vi "Calculate Dynamic VariablesA.vi"(7 "Frequencies":dbl[](array[numeric]), 8 "Hours Under Test":dbl[](array[numeric]), 9 "Nom Freq":string) -> (0 "Agerate1Y":dbl, 1 "Agerate30D":dbl, 2 "C":dbl, 3 "B":dbl, 4 "RMS":dbl, 5 "A":dbl)   [LabVIEW 2024]
panel:
  out "Base ppm":dbl
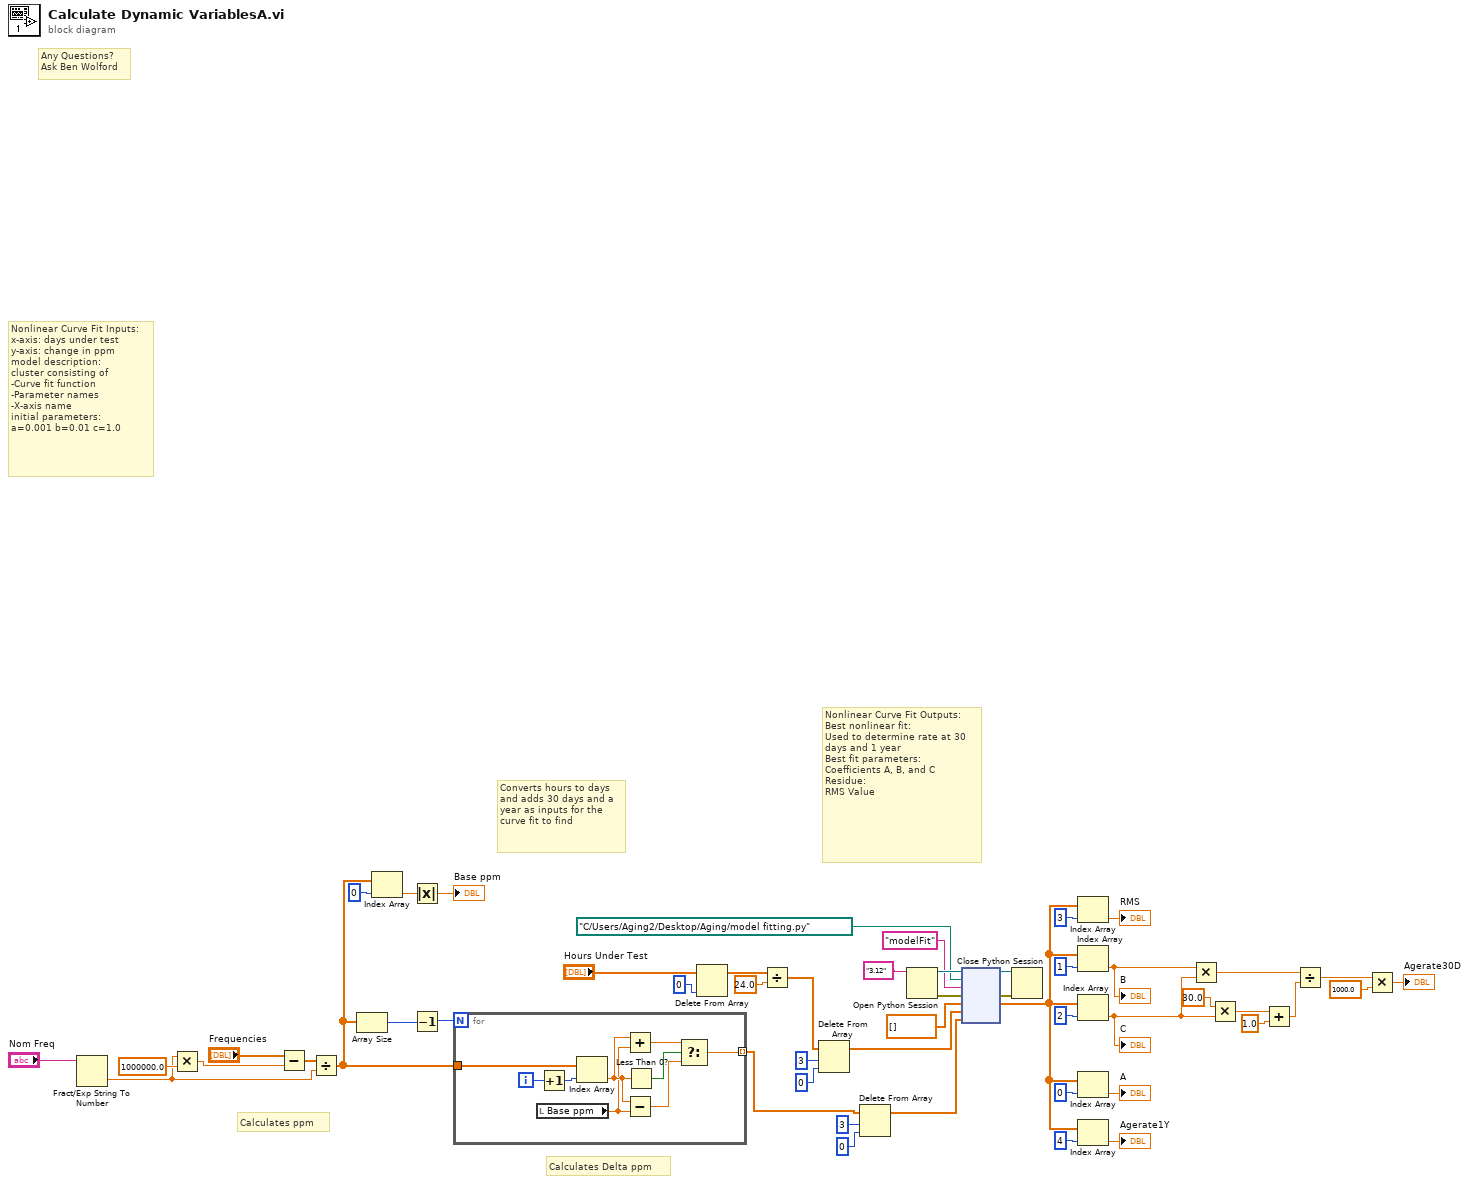
[diagram p0: block diagram]
diagram:
  # "Any Questions?\nAsk Ben Wolford"
  # "Calculates Delta ppm"
  # "Converts hours to days and adds 30 days and a year as inputs for the curve fit to find"
  # "Calculates ppm"
  # "Nonlinear Curve Fit Outputs:\nBest nonlinear fit:\nUsed to determine rate at 30 days and 1 year\nBest fit parameters:\nCoefficients A, B, and C\nResidue:\nRMS Value"
  # "Nonlinear Curve Fit Inputs:\nx-axis: days under test\ny-axis: change in ppm \nmodel description:\ncluster consisting of\n-Curve fit function\n-Parameter names\n-X-axis name\ninitial parameters:\na=0.001 b=0.01 c=1.0"
  n1 = Fract/Exp String To Number(string="Nom Freq") -> (number=w47:dbl)  [unwired: 3 in, 1 out]
  n2 = Multiply(x=w47, y=1000000.0) -> (x*y=w38:dbl)
  n3 = Subtract(x="Frequencies", y=w38) -> (x-y=w48:dbl[])
  n4 = Divide(x=w48, y=w47) -> (x/y=w43:dbl[])
  n5 = Array Size(array=w43) -> (size(s)=w45:i32)
  n6 = Index Array(array=w43, index=0) -> (element=w37:dbl)
  n7 = Absolute Value(x=w37) -> (abs(x)=→"Base ppm":dbl)
  n8 = Decrement(x=w45) -> (x-1=w44:i32)
  n9 = for {
    N: w44 -> [_]
    tunnel: w43 -> [w58]
    tunnel: [w55] -> w6 mode=indexing
    i -> [w59]
    n10 = local read "Base ppm"() -> (w53:dbl)
    n11 = Increment(x=w59) -> (x+1=w60:i32)
    n12 = Index Array(array=w58, index=w60) -> (element=w54:dbl)
    n13 = Add(x=w54, y=w53) -> (x+y=w52:dbl)
    n14 = Subtract(x=w54, y=w53) -> (x-y=w56:dbl)
    n15 = Less Than 0?(x=w54) -> (x < 0?=w57:bool)
    n16 = Select(t=w52, s=w57, f=w56) -> (s? t:f=w55:dbl)
  }
  n17 = Delete From Array(array="Hours Under Test", index=0) -> (array with subset deleted=w40:dbl[])  [unwired: 1 in, 1 out]
  n18 = Divide(x=w40, y=24.0) -> (x/y=w2:dbl[])
  n19 = Delete From Array(array=w2, length=3, index=0) -> (array with subset deleted=w1:dbl[])  [unwired: 1 out]
  n20 = Delete From Array(array=w6, length=3, index=0) -> (array with subset deleted=w5:dbl[])  [unwired: 1 out]
  n21 = Open Python Session(python version="3.12" ("Python version")) -> (session out=w25:refnum<k35>, error out=w26:errorcluster)  [unwired: 2 in]
  n22 = node ("Python Node")(w25, path "C:/Users/Aging2/Desktop/Aging/model fitting.py" ("module path"), "modelFit" ("function name"), w26, dbl[] [], w1, w5) -> (w23:refnum<k35>, w24:errorcluster, w14:dbl[])  [unwired: 2 in, 2 out]
  n23 = Close Python Session(session in=w23, error in=w24) -> ()  [unwired: 1 out]
  n24 = Index Array(array=w14, index=3) -> (element=→"RMS":dbl)
  n25 = Index Array(array=w14, index=1) -> (element=w10:dbl)
  "B" <- w10
  n26 = Index Array(array=w14, index=2) -> (element=w9:dbl)
  "C" <- w9
  n27 = Index Array(array=w14, index=0) -> (element=→"A":dbl)
  n28 = Index Array(array=w14, index=4) -> (element=→"Agerate1Y":dbl)
  n29 = Multiply(x=w10, y=w9) -> (x*y=w31:dbl)
  n30 = Multiply(x=30.0, y=w9) -> (x*y=w34:dbl)
  n31 = Add(x=w34, y=1.0) -> (x+y=w32:dbl)
  n32 = Divide(x=w31, y=w32) -> (x/y=w30:dbl)
  n33 = Multiply(x=w30, y=1000.0) -> (x*y=→"Agerate30D":dbl)
